vi "OpenTIFF.vi"(8 "error in (no error)":errorcluster, 10 "Opening Purpose":T1, 11 "File Path":path) -> (0 "error out":errorcluster, 3 "TIFF File Ref":i32)   [LabVIEW 2012]
uses:
  Opening Purpose.ctl
  VisualCPP/LabTIFF/Release/LabTIFF.dll
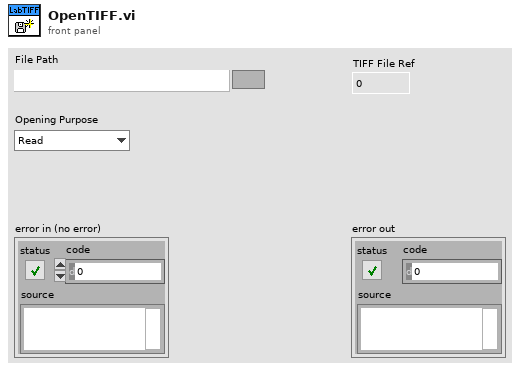
[diagram p1: front panel]
types:
  T1 = typedef "Opening Purpose.ctl" = enum16{"Read", "Write"}
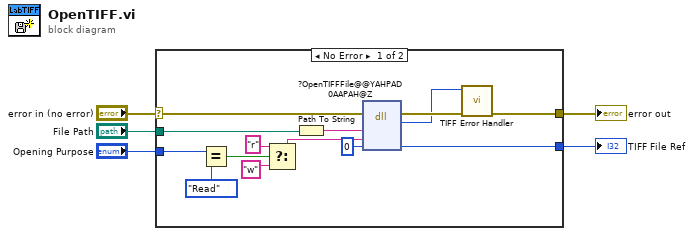
[diagram p0: block diagram]
diagram:
  n1 = case shown="No Error" "error in (no error)" {
    selector: "error in (no error)" -> [w19 w20]
    tunnel: "File Path" -> [w18 _]
    tunnel: "Opening Purpose" -> [w16 _]
    tunnel: [w9 _] -> w2
    tunnel: [w6 w20] -> w1
    frame No Error {
      n2 = Equal?(x=w16, y=Opening_Purpose."Read") -> (x = y?=w14:bool)
      n3 = Select(t="r", s=w14, f="w") -> (s? t:f=w11:string)
      n4 = Path To String(path=w18) -> (string=w17:string)
      n5 = dll-call lib="C:/Users/Ludovico/Prog/moroder/dependencies/LabTIFF/VisualCPP/LabTIFF/Release/LabTIFF.dll" fn="?OpenTIFFFile@@YAHPAD0AAPAH@Z"(error in=w19, "Path"=w17, "Opening Purpose"=w11, "File Reference"=0) -> (error out=w8:errorcluster, "Error"=w7:i32, "File Reference"=w9:i32)  [unwired: 4 in, 1 out]
      n6 = call "TIFF Error Handler.vi"("error in (no error)"=w8, "TIFF DLL error"=w7) -> ("error out"=w6:errorcluster)  [unwired: 9 in]
    }
    frame Error {
    }
  }
  "TIFF File Ref" <- w2
  "error out" <- w1
